vi "SeimensS7Net_ReadString.vi"(8 "error in (no error)":errorcluster caption="错误输入（无错误）", 10 "address":string="DB600.0", 11 "Seimens 输入":refnum<class "Seimens.lvclass">) -> (0 "error out":errorcluster caption="错误输出", 2 "Content":string, 3 "Seimens 输出":refnum<class "Seimens.lvclass">)   [LabVIEW 2018, in "Seimens.lvclass"]
uses:
  Seimens.lvclass
  Seimens.lvclass/Seimens.ctl
  D:/LiMing/Labview/lib/LM_HslCommunication/DLL/HslCommunication.dll
  DLL/HslCommunication.dll
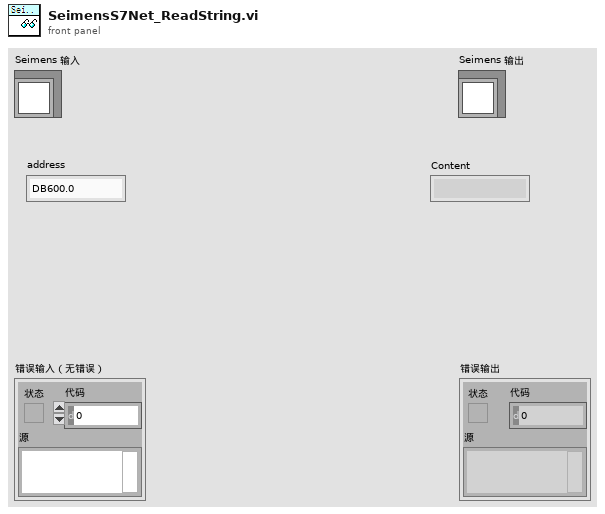
[diagram p1: front panel]
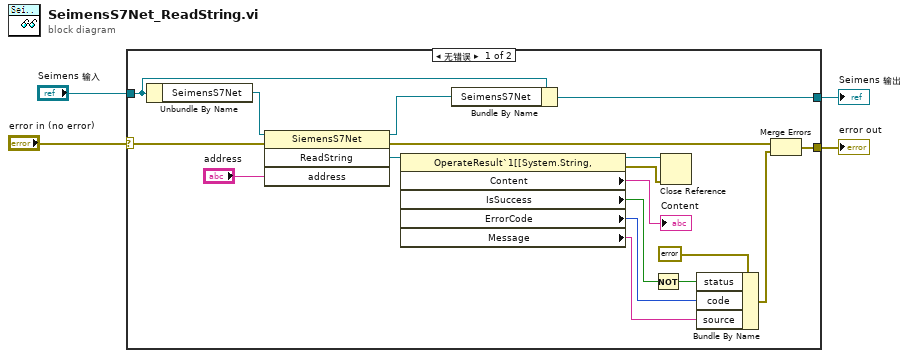
[diagram p0: block diagram]
diagram:
  n1 = case shown="无错误" "error in (no error)" {
    selector: "error in (no error)" -> [w8 w24]
    tunnel: [w7 w24] -> w3
    tunnel: [w10 w23] -> w1
    tunnel: "Seimens 输入" -> [w11 w23]
    frame No Error {
      n2 = Unbundle By Name(w11) -> ("SeimensS7Net"=w12:refnum<k24>)
      n3 = invoke class="SiemensS7Net" method="ReadString"(reference=w12, error in=w8, "address"="address") -> (reference out=w9:refnum<k24>, error out=w18:errorcluster, "ReadString"=w15:refnum<k24>)  [unwired: 1 in, 1 out]
      n4 = property class="OperateResult`1[[System.String,"(reference=w15) -> (reference out=w17:refnum<k24>, error out=w16:errorcluster, "Content"=→"Content":string, "IsSuccess"=w19:bool, "ErrorCode"=w20:i32, "Message"=w21:string)  [unwired: 1 in]
      n5 = Bundle By Name(cluster=w11, "SeimensS7Net"=w9) -> (w10:refnum<class "Seimens.lvclass">)
      n6 = Not(x=w19) -> (.not. x?=w5:bool)
      n7 = Close Reference(reference=w17, error in (no error)=w16) -> ()  [unwired: 1 out]
      n8 = Bundle By Name(cluster=errorcluster {"status"=FALSE, "code"=0, "source"=""} ("error in (no error)"), "status"=w5, "code"=w20, "source"=w21) -> (w22:errorcluster)
      n9 = Merge Errors(w18, w22) -> (w7:errorcluster)
    }
    frame Error {
    }
  }
  "error out" <- w3
  "Seimens 输出" <- w1
